vi "Reset.vi"(8 "error in (no error)":errorcluster, 9 "channel (1)":u8=1 min=1 max=4 step=1, 10 "reset (T:device)":bool=TRUE, 11 "VISA resource name":refnum<visa-resource-name>) -> (0 "error out":errorcluster, 3 "VISA resource name out":refnum<visa-resource-name>)   [LabVIEW 2020, in "Agilent 6XXX Series.lvlib"]
doc: "This VI resets the instrument or resets the output after the instrument trips the OVP or OCP. Consult the user's manual for the default parameter settings to which this command resets the instrument."
uses:
  <instrlib>/Agilent 6XXX Series/Agilent 6XXX Series.lvlib
panel:
  # "device\nOV/OC"
  # "*662xA only"
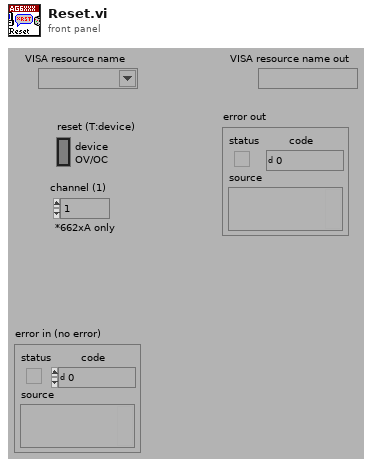
[diagram p1: front panel]
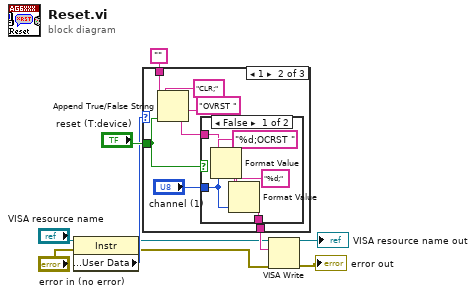
[diagram p0: block diagram]
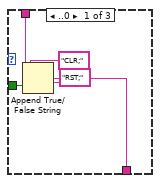
[diagram p2: hidden frame]
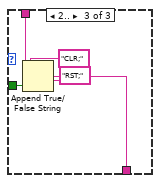
[diagram p4: hidden frame]
diagram:
  n1 = property class="Instr"(reference="VISA resource name", error in="error in (no error)") -> (reference out=w4:refnum<visa-resource-name>, error out=w3:errorcluster, "General Settings:User Data"=w5:u32)
  n2 = case shown="1" w5 {
    tunnel: "" -> [w13 w20 w32]
    tunnel: "reset (T:device)" -> [w12 w19 w31]
    tunnel: [w11 w16 w30] -> w6
    frame ..0 {
      n3 = Append True/False String(1:w12, 2:"RST;", 3:"CLR;" ("Reset Command"), 4:w13) -> (0:w11:string)
    }
    frame 1 {
      n4 = Append True/False String(1:w19, 2:"OVRST ", 3:"CLR;" ("Reset Command"), 4:w20) -> (0:w18:string)
      n5 = case shown="False" w19 {
        tunnel: w18 -> [w25 w29]
        tunnel: "channel (1)" -> [w24 _]
        tunnel: [w23 w29] -> w16
        frame False {
          n6 = Format Value(string ("")=w25, format string="%d;OCRST ", value (0)=w24) -> (output string=w27:string)
          n7 = Format Value(string ("")=w27, format string="%d;", value (0)=w24) -> (output string=w23:string)
        }
        frame True {
        }
      }
    }
    frame 2.. {
      n8 = Append True/False String(1:w31, 2:"RST;", 3:"CLR;" ("Reset Command"), 4:w32) -> (0:w30:string)
    }
  }
  n9 = VISA Write(VISA resource name=w4, write buffer=w6, error in (no error)=w3) -> (VISA resource name out=→"VISA resource name out":refnum<visa-resource-name>, error out=→"error out":errorcluster)  [unwired: 1 out]
